vi "Calcolo Errori 2.vi"(10 "Misure":T3, 11 "Riferimenti":T2) -> (0 "TVE":waveform(dbl)(graph), 1 "Errore Frequenza":waveform(dbl)(graph), 2 "Errore Fase":waveform(dbl)(graph), 3 "Errore Ampiezza":waveform(dbl)(graph), 4 "Frequenza Misurata":waveform(dbl)[](graph), 5 "Fase Misurata":waveform(dbl)[](graph), 7 "Ampiezza Misurata":waveform(dbl)[](graph))   [LabVIEW 2019]
uses:
  <vilib>/Analysis/coordinate.llb/Wrap Angle (scalar).vi
  <vilib>/Analysis/NI_AAL_Angle.lvlib
panel:
  in  "Tab Control":T1(tab)
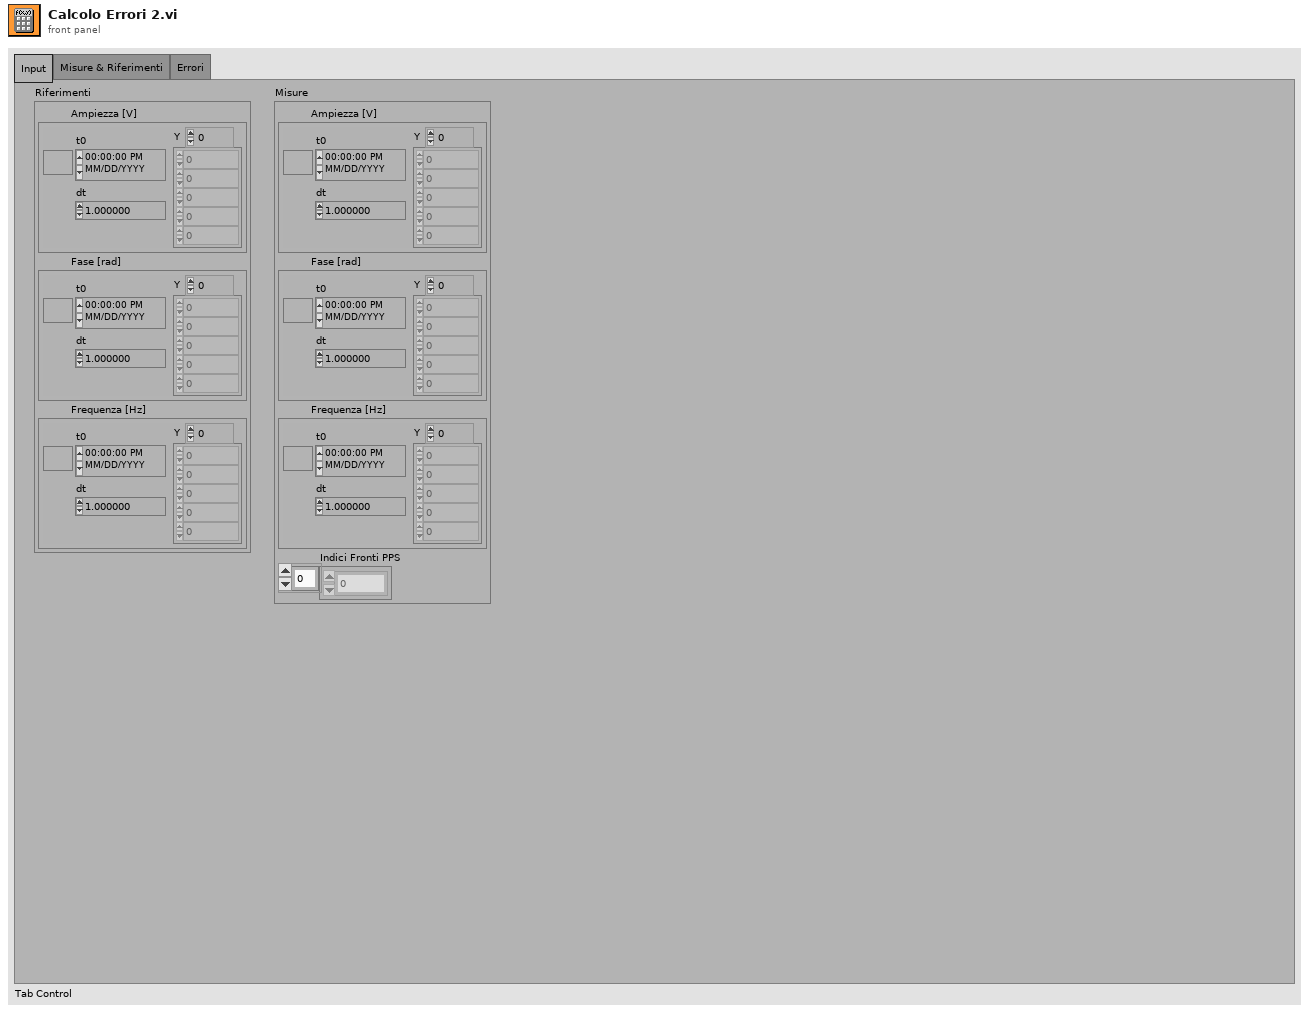
[diagram p1: front panel]
types:
  T1 = enum32{"Input", "Misure & Riferimenti", "Errori"}
  T2 = cluster{"Ampiezza [V]":waveform(dbl), "Fase [rad]":waveform(dbl), "Frequenza [Hz]":waveform(dbl)}
  T3 = cluster{"Ampiezza [V]":waveform(dbl), "Fase [rad]":waveform(dbl), "Frequenza [Hz]":waveform(dbl), "Indici Fronti PPS":i32[]}
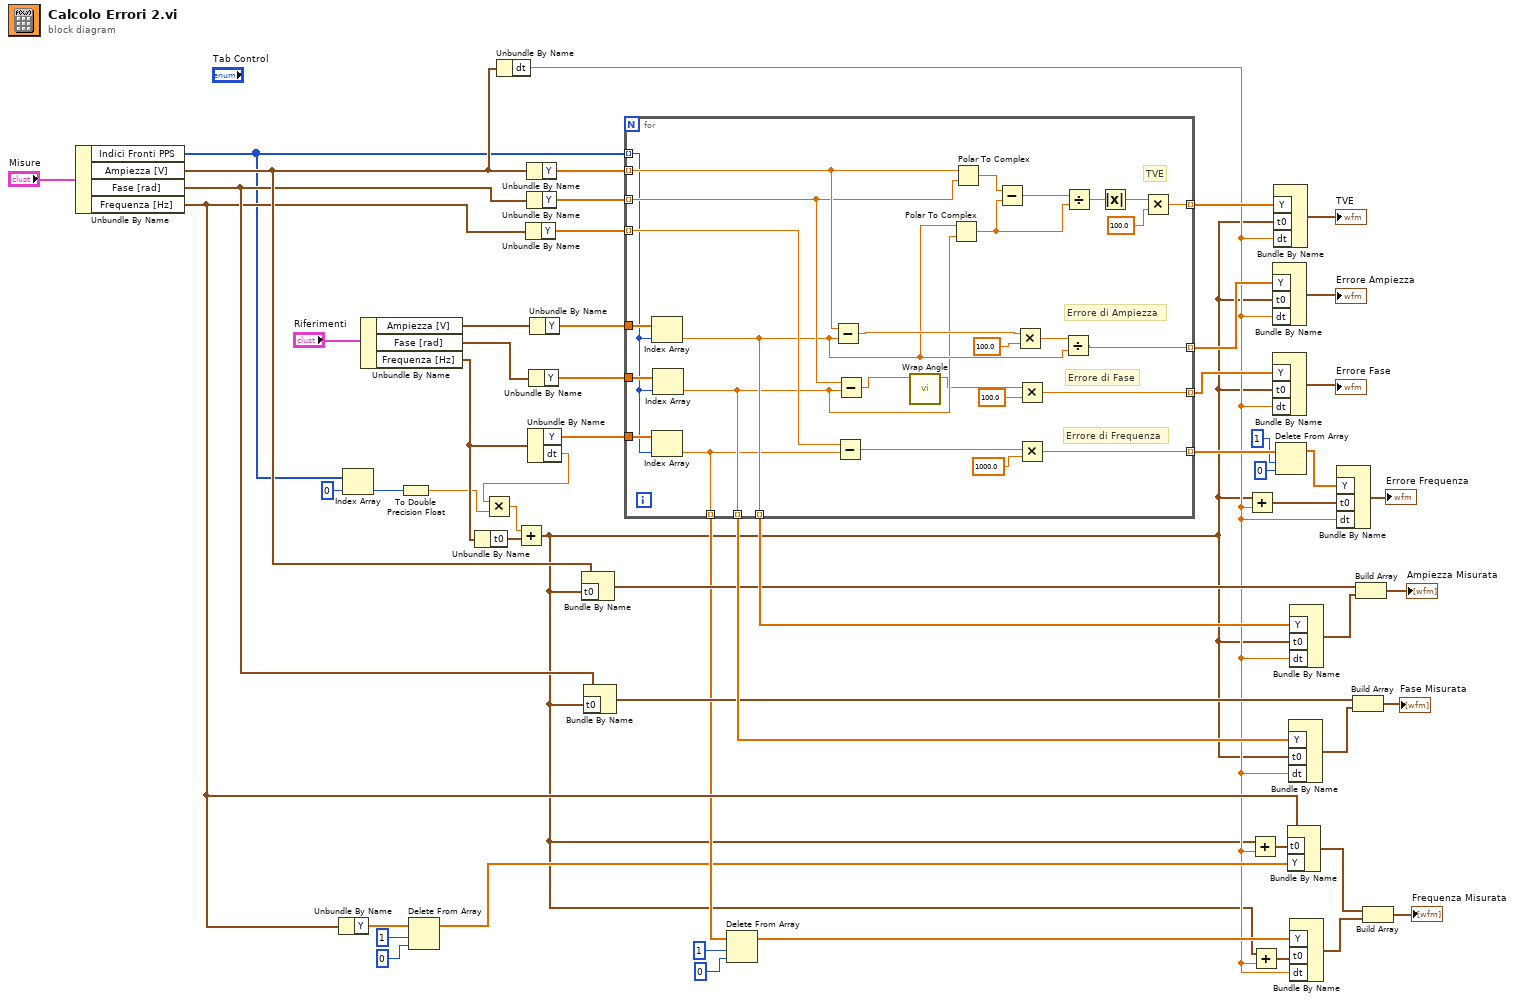
[diagram p0: block diagram]
diagram:
  n1 = Unbundle By Name "Unbundle By Name"("Misure") -> ("Indici Fronti PPS"=w8:i32[], "Ampiezza [V]"=w33:waveform(dbl), "Fase [rad]"=w32:waveform(dbl), "Frequenza [Hz]"=w20:waveform(dbl))
  n2 = Unbundle By Name(w20) -> ("Y"=w19:dbl[])
  n3 = Index Array "Index Array"(array=w8, index=0) -> (element=w4:i32)
  n4 = Unbundle By Name "Unbundle By Name"("Riferimenti") -> ("Ampiezza [V]"=w52:waveform(dbl), "Fase [rad]"=w54:waveform(dbl), "Frequenza [Hz]"=w51:waveform(dbl))
  n5 = To Double Precision Float(number=w4) -> (double precision float=w2:dbl)
  n6 = Delete From Array "Delete From Array"(array=w19, length=1, index=0) -> (array with subset deleted=w12:dbl[])  [unwired: 1 out]
  n7 = Unbundle By Name(w51) -> ("t0"=w7:timestamp)
  n8 = Unbundle By Name ("Get Waveform Components")(w33) -> ("dt"=w10:dbl)
  n9 = Unbundle By Name(w20) -> ("Y"=w53:dbl[])
  n10 = Unbundle By Name(w33) -> ("Y"=w40:dbl[])
  n11 = Unbundle By Name(w32) -> ("Y"=w39:dbl[])
  n12 = Unbundle By Name(w51) -> ("Y"=w38:dbl[], "dt"=w3:dbl)
  n13 = Multiply(x=w3, y=w2) -> (x*y=w1:dbl)
  n14 = Add(x=w1, y=w7) -> (x+y=w6:timestamp)
  n15 = Unbundle By Name(w54) -> ("Y"=w41:dbl[])
  n16 = Unbundle By Name(w52) -> ("Y"=w42:dbl[])
  n17 = Bundle By Name(cluster=w33, "t0"=w6) -> (w26:waveform(dbl))
  n18 = Bundle By Name(cluster=w32, "t0"=w6) -> (w24:waveform(dbl))
  n19 = for {
    tunnel: w42 -> [w84]
    tunnel: w40 -> [w65] mode=indexing
    tunnel: w41 -> [w83]
    tunnel: w38 -> [w82]
    tunnel: w39 -> [w64] mode=indexing
    tunnel: w53 -> [w63] mode=indexing
    tunnel: w8 -> [w59] mode=indexing
    tunnel: [w76] -> w50 mode=indexing
    tunnel: [w66] -> w49 mode=indexing
    tunnel: [w71] -> w48 mode=indexing
    tunnel: [w69] -> w31 mode=indexing
    tunnel: [w62] -> w36 mode=indexing
    tunnel: [w61] -> w37 mode=indexing
    tunnel: [w60] -> w16 mode=indexing
    # "TVE"
    # "Errore di Frequenza"
    # "Errore di Fase"
    # "Errore di Ampiezza"
    n20 = Index Array "Index Array"(array=w84, index=w59) -> (element=w62:dbl)
    n21 = Index Array "Index Array"(array=w82, index=w59) -> (element=w60:dbl)
    n22 = Index Array "Index Array"(array=w83, index=w59) -> (element=w61:dbl)
    n23 = Subtract(x=w65, y=w62) -> (x-y=w74:dbl)
    n24 = Subtract(x=w63, y=w60) -> (x-y=w70:dbl)
    n25 = Subtract(x=w64, y=w61) -> (x-y=w58:dbl)
    n26 = call-poly <vilib>:"Wrap Angle.vi"("angle in"=w58) -> ("angle out"=w57:dbl)  [unwired: 9 in, 1 out]
    n27 = Polar To Complex(1:w61, 2:w62) -> (0:w79:cdb)
    n28 = Polar To Complex(1:w64, 2:w65) -> (0:w81:cdb)
    n29 = Subtract(x=w81, y=w79) -> (x-y=w80:cdb)
    n30 = Multiply(x=w74, y=100.0) -> (x*y=w67:dbl)
    n31 = Multiply(x=w57, y=100.0) -> (x*y=w71:dbl)
    n32 = Multiply(x=w70, y=1000.0) -> (x*y=w69:dbl)
    n33 = Divide(x=w67, y=w62) -> (x/y=w66:dbl)
    n34 = Divide(x=w80, y=w79) -> (x/y=w78:cdb)
    n35 = Absolute Value(x=w78) -> (abs(x)=w77:dbl)
    n36 = Multiply(x=w77, y=100.0) -> (x*y=w76:dbl)
  }
  n37 = Delete From Array "Delete From Array"(array=w16, length=1, index=0) -> (array with subset deleted=w11:dbl[])  [unwired: 1 out]
  n38 = Add(x=w6, y=w10) -> (x+y=w43:timestamp)
  n39 = Add(x=w6, y=w10) -> (x+y=w9:timestamp)
  n40 = Add(x=w6, y=w10) -> (x+y=w13:timestamp)
  n41 = Bundle By Name("Y"=w49, "t0"=w6, "dt"=w10) -> (→"Errore Ampiezza":waveform(dbl))  [unwired: 1 in]
  n42 = Bundle By Name("Y"=w48, "t0"=w6, "dt"=w10) -> (→"Errore Fase":waveform(dbl))  [unwired: 1 in]
  n43 = Bundle By Name("Y"=w50, "t0"=w6, "dt"=w10) -> (→"TVE":waveform(dbl))  [unwired: 1 in]
  n44 = Delete From Array "Delete From Array"(array=w31, length=1, index=0) -> (array with subset deleted=w28:dbl[])  [unwired: 1 out]
  n45 = Bundle By Name(cluster=w20, "t0"=w9, "Y"=w12) -> (w23:waveform(dbl))
  n46 = Bundle By Name("Y"=w37, "t0"=w6, "dt"=w10) -> (w25:waveform(dbl))  [unwired: 1 in]
  n47 = Bundle By Name("Y"=w36, "t0"=w6, "dt"=w10) -> (w27:waveform(dbl))  [unwired: 1 in]
  n48 = Bundle By Name("Y"=w11, "t0"=w13, "dt"=w10) -> (w21:waveform(dbl))  [unwired: 1 in]
  n49 = Bundle By Name("Y"=w28, "t0"=w43, "dt"=w10) -> (→"Errore Frequenza":waveform(dbl))  [unwired: 1 in]
  n50 = Build Array(w24, w25) -> (→"Fase Misurata":waveform(dbl)[])
  n51 = Build Array(w26, w27) -> (→"Ampiezza Misurata":waveform(dbl)[])
  n52 = Build Array(w23, w21) -> (→"Frequenza Misurata":waveform(dbl)[])
